vi "Get Actor Details.vi"(0 "Application":refnum<vi>, 5 "Method Qualified Name":string, 11 "error in (no error)":errorcluster) -> (4 "Actor Name":string, 6 "Actor Path":path, 8 "Actor Method VI Reference":refnum<vi>, 10 "Actor Reference":refnum<vi>, 15 "error out":errorcluster)   [LabVIEW 2023, in "Message Maker.lvclass"]
doc: "Gets the Actor path, name and VI Server reference from the Method FQN"
uses:
  Message Maker.lvclass
  Message Maker.lvclass/Message Maker.ctl
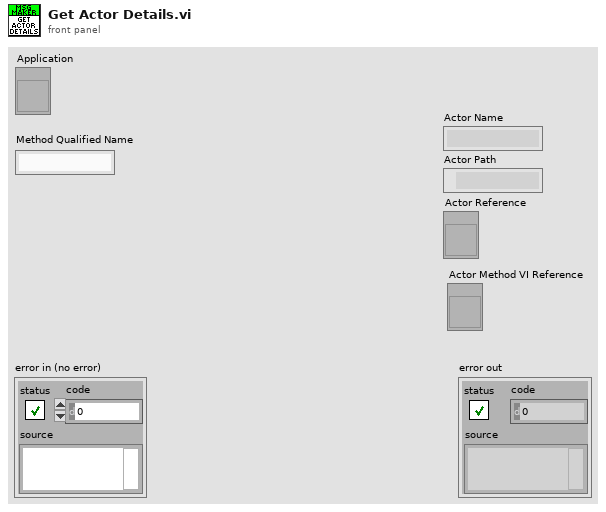
[diagram p1: front panel]
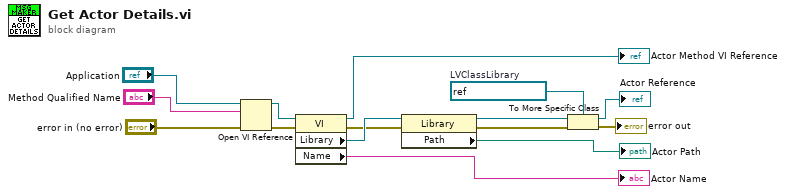
[diagram p0: block diagram]
diagram:
  w11 = refnum<vi> refnum  # LVClassLibrary
  n1 = Open VI Reference(application reference (local)="Application", vi path="Method Qualified Name", error in (no error)="error in (no error)") -> (vi reference=w14:refnum<vi>, error out=w15:errorcluster)  [unwired: 3 in]
  n2 = property class="VI"(reference=w14, error in=w15) -> (reference out=→"Actor Method VI Reference":refnum<vi>, error out=w9:errorcluster, "Library"=w13:refnum<vi>, "Name"=→"Actor Name":string)
  n3 = property class="Library"(reference=w13, error in=w9) -> (reference out=w12:refnum<vi>, error out=w8:errorcluster, "Path"=→"Actor Path":path)
  n4 = To More Specific Class(target class=w11, reference=w12, error in=w8) -> (specific class reference=→"Actor Reference":refnum<vi>, error out=→"error out":errorcluster)
